vi "ShooterLookup.vi"(8 "Shooter Speeds":cluster{"Distance":sgl, "Speed":sgl}[](array[cluster])=[{"Distance"=0.0, "Speed"=2800.0}, {"Distance"=107.0, "Speed"=2800.0}, {"Distance"=162.0, "Speed"=3700.0}, {"Distance"=185.0, "Speed"=3700.0}, {"Distance"=195.0, "Speed"=3700.0}, {"Distance"=300.0, "Speed"=4200.0}], 11 "Distance":dbl) -> (1 "Elevation":bool, 3 "Speed":dbl)   [LabVIEW 2011]
uses:
  Robot Global Data.vi
panel:
  in  "Squish Lookup":cluster{"Squish":sgl, "Factor":sgl}[](array[cluster])=[{"Squish"=0.0, "Factor"=1.0}, {"Squish"=3.79, "Factor"=1.0}, {"Squish"=3.87, "Factor"=0.971}, {"Squish"=3.89, "Factor"=0.953}, {"Squish"=3.91, "Factor"=0.914}, {"Squish"=5.0, "Factor"=0.914}]
  in  "Cluster":T1={"Shooter"=1850.0, "Override"=FALSE, "Inclenation"=FALSE}
  in  "Elevation TH":dbl=120.0
  # "28 = front to fender\n54.75 = back to fender\n160 = key"
  # "Use these values\nRather than Lookup"
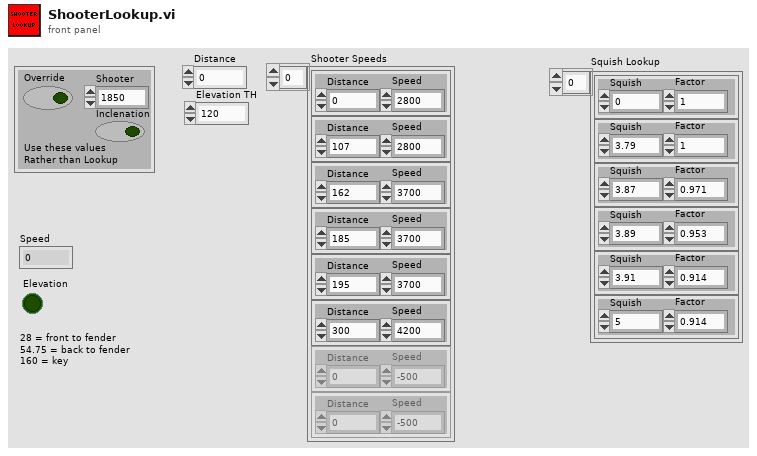
[diagram p1: front panel]
types:
  T1 = cluster{"Shooter":dbl, "Override":bool, "Inclenation":bool}
  T2 = typedef "Position Typedef.ctl" = cluster{"X":dbl, "Y":dbl, "Heading":dbl}
  T3 = typedef "Target Typedef.ctl" = cluster{"X":dbl, "Y":dbl, "Deltax":dbl, "Distance":dbl}
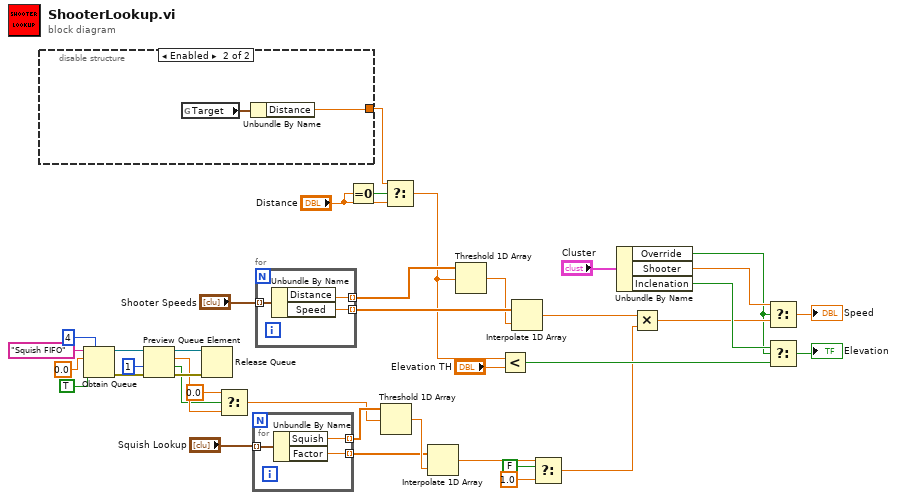
[diagram p0: block diagram]
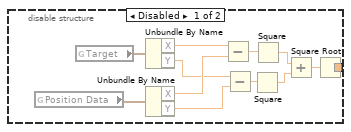
[diagram p2: hidden frame]
diagram:
  n1 = disable-structure shown="Enabled" {
    disable-tunnel: [w51 w52] -> w33
    frame Disabled {
      n2 = global read "Robot Global Data.vi" "Position Data"() -> (w41:T2)
      n3 = global read "Robot Global Data.vi" "Target"() -> (w40:T3)
      n4 = Unbundle By Name(w40) -> ("X"=w42:dbl, "Y"=w43:dbl)
      n5 = Unbundle By Name(w41) -> ("X"=w44:dbl, "Y"=w45:dbl)
      n6 = Subtract(x=w42, y=w44) -> (x-y=w46:dbl)
      n7 = Subtract(x=w43, y=w45) -> (x-y=w47:dbl)
      n8 = Square(x=w47) -> (x^2=w48:dbl)
      n9 = Square(x=w46) -> (x^2=w49:dbl)
      n10 = Add(x=w49, y=w48) -> (x+y=w50:dbl)
      n11 = Square Root(x=w50) -> (sqrt(x)=w51:dbl)
    }
    frame Enabled {
      n12 = global read "Robot Global Data.vi" "Target"() -> (w53:T3)
      n13 = Unbundle By Name(w53) -> ("Distance"=w52:dbl)
    }
  }
  n14 = Obtain Queue(max queue size (-1, unlimited)=4, name (unnamed)="Squish FIFO", element data type=sgl 0.0 ("Voltage"), create if not found? (T)=TRUE) -> (queue out=w10:refnum<queue>, error out=w11:errorcluster)  [unwired: 1 in, 1 out]
  n15 = Preview Queue Element(queue=w10, timeout in ms (-1)=1, error in (no error)=w11) -> (queue out=w6:refnum<queue>, element=w3:sgl, timed out?=w2:bool, error out=w7:errorcluster)
  n16 = Release Queue(queue=w6, error in (no error)=w7) -> ()  [unwired: 1 in, 3 out]
  n17 = Select(t=0.0, s=w2, f=w3) -> (s? t:f=w1:dbl)
  n18 = for {
    tunnel: "Squish Lookup" -> [w56] mode=indexing
    tunnel: [w55] -> w24 mode=indexing
    tunnel: [w54] -> w22 mode=indexing
    n19 = Unbundle By Name(w56) -> ("Squish"=w55:sgl, "Factor"=w54:sgl)
  }
  n20 = for {
    tunnel: "Shooter Speeds" -> [w59] mode=indexing
    tunnel: [w58] -> w38 mode=indexing
    tunnel: [w57] -> w37 mode=indexing
    n21 = Unbundle By Name(w59) -> ("Distance"=w58:sgl, "Speed"=w57:sgl)
  }
  n22 = Equal To 0?(x="Distance") -> (x = 0?=w34:bool)
  n23 = Threshold 1D Array(2:w1, 3:w24) -> (0:w23:sgl)  [unwired: 1 in]
  n24 = Select(t=w33, s=w34, f="Distance") -> (s? t:f=w31:dbl)
  n25 = Interpolate 1D Array(1:w23, 2:w22) -> (0:w21:sgl)
  n26 = Threshold 1D Array(2:w31, 3:w38) -> (0:w36:sgl)  [unwired: 1 in]
  n27 = Less?(x=w31, y="Elevation TH") -> (x < y?=w28:bool)
  n28 = Interpolate 1D Array(1:w36, 2:w37) -> (0:w16:sgl)
  n29 = Select(t=w21, s=FALSE, f=sgl 1.0) -> (s? t:f=w20:sgl)
  n30 = Unbundle By Name("Cluster") -> ("Override"=w14:bool, "Shooter"=w15:dbl, "Inclenation"=w30:bool)
  n31 = Multiply(x=w16, y=w20) -> (x*y=w17:sgl)
  n32 = Select(t=w15, s=w14, f=w17) -> (s? t:f=→"Speed":dbl)
  n33 = Select(t=w30, s=w14, f=w28) -> (s? t:f=→"Elevation":bool)
